vi "Get Optimiser Configuration as string.vi"(8 "error in (no error)":errorcluster, 11 "Optimiser Cell in":refnum<class "Optimiser Cell.lvclass">) -> (0 "error out":errorcluster, 2 "Info":string, 3 "Optimiser Cell out":refnum<class "Optimiser Cell.lvclass">)   [LabVIEW 2020, in "CIRCUS_uServices.lvlib" / "Run Utilities.lvlib" / "Optimiser Cell.lvclass"]
uses:
  Optimiser Cell.lvclass
  Optimiser Cell.lvclass/Optimiser Cell.ctl
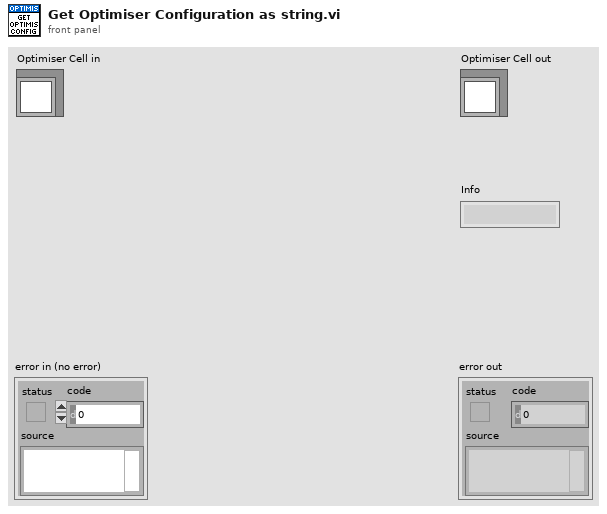
[diagram p1: front panel]
types:
  T1 = typedef "CIRCUS_uServices.lvlib/Run Utilities.lvlib/Optimiser Cell.lvclass/Optimise parameter - numeric.ctl" = cluster{"Name":string, "Start value":dbl, "From":dbl, "To":dbl, "dtype":enum16{"INT", "DBL"}}
  T2 = typedef "CIRCUS_uServices.lvlib/Run Utilities.lvlib/Optimiser Cell.lvclass/Optimise parameter - string.ctl" = cluster{"Name":string, "Start value":string, "Options":string[]}
  T3 = typedef "CIRCUS_uServices.lvlib/Run Utilities.lvlib/Optimiser Cell.lvclass/Optimisation observable.ctl" = cluster{"Name":string, "Weight":dbl}
  T4 = typedef "CIRCUS_uServices.lvlib/Run Utilities.lvlib/Optimiser Cell.lvclass/Optimisation Strategy.ctl" = enum16{"Maximize", "Minimize", "Value"}
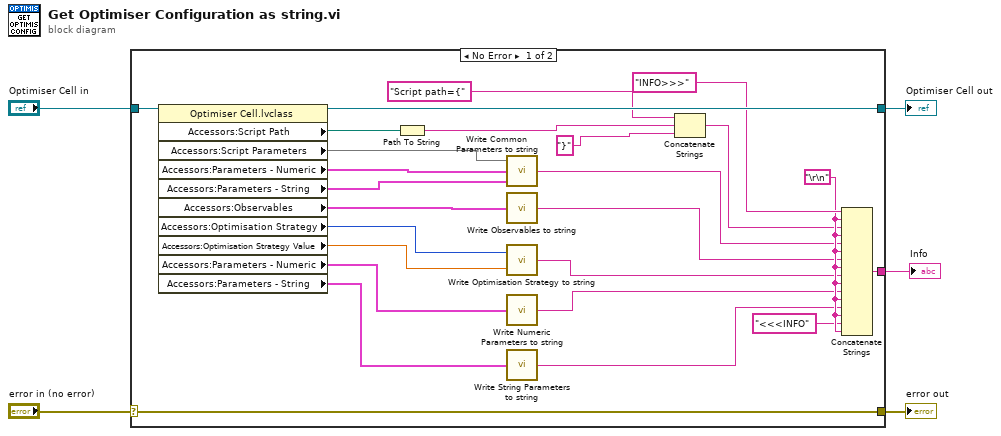
[diagram p0: block diagram]
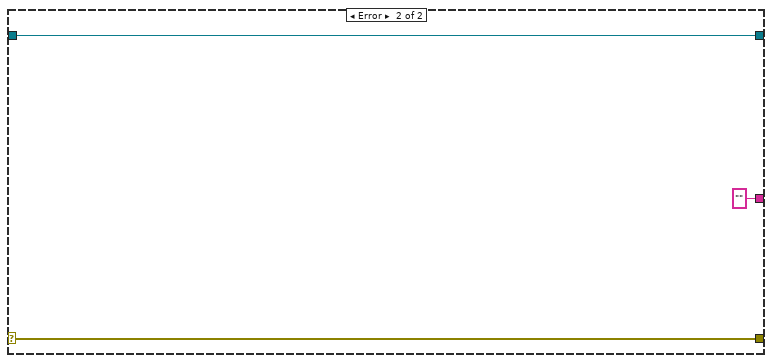
[diagram p2: hidden frame]
diagram:
  n1 = case shown="No Error" "error in (no error)" {
    selector: "error in (no error)" -> [w30 w33]
    tunnel: [w30 w33] -> w4
    tunnel: [w29 w32] -> w2
    tunnel: "Optimiser Cell in" -> [w22 w32]
    tunnel: [w20 ""] -> w1
    frame No Error {
      w24 = "\r\n"
      n2 = property class="Optimiser Cell.lvclass"(reference=w22) -> (reference out=w29:refnum<class "Optimiser Cell.lvclass">, "Accessors:Script Path"=w27:path, "Accessors:Script Parameters"=w16:map{string, string}, "Accessors:Parameters - Numeric"=w15:T1[], "Accessors:Parameters - String"=w14:T2[], "Accessors:Observables"=w11:T3[], "Accessors:Optimisation Strategy"=w8:T4, "Accessors:Optimisation Strategy Value"=w7:dbl, "Accessors:Parameters - Numeric"=w10:T1[], "Accessors:Parameters - String"=w9:T2[])  [unwired: 1 in, 1 out]
      n3 = Path To String(path=w27) -> (string=w26:string)
      n4 = call "Write Common Parameters to string.vi"("Parameters - String"=w14, "Parameters - Numeric"=w15, "Script Parameters"=w16) -> ("String"=w13:string)
      n5 = call "Write Observables to string.vi"("Observables"=w11) -> ("String"=w17:string)
      n6 = call "Write Optimisation Strategy to string.vi"("Value"=w7, "Optimisation Strategy"=w8) -> ("String"=w6:string)
      n7 = call "Write Numeric Parameters to string.vi"("Parameters - numeric"=w10) -> ("String"=w19:string)
      n8 = call "Write String Parameters to string.vi"("Parameters - string"=w9) -> ("String"=w18:string)
      n9 = Concatenate Strings("Script path={" ("string"), w26, "}" ("string")) -> (w23:string)
      n10 = Concatenate Strings("INFO>>>" ("string"), w24, w23, w24, w13, w24, w17, w24, w6, w24, w19, w24, w18, w24, "<<<INFO" ("string"), w24) -> (w20:string)
    }
    frame Error {
    }
  }
  "error out" <- w4
  "Optimiser Cell out" <- w2
  "Info" <- w1
